vi "Load Proto File.vi"(8 "error in (no error)":errorcluster, 10 "Proto File Path":path, 11 "OOP Server in":refnum<class "Template Server.lvclass">) -> (0 "error out":errorcluster, 3 "OOP Server out":refnum<class "Template Server.lvclass">)   [LabVIEW 2019, in "Template Server.lvlib" / "Template Server.lvclass"]
uses:
  Template Server.lvclass
  typeDefs/Server gRPC UEs.ctl
  gRPC interface/Server API/typeDefs/Message Metadata.ctl
  gRPC interface/Server API/typeDefs/Message Element Metadata.ctl
  gRPC interface/Server API/typeDefs/Message Element Type.ctl
  typeDefs/Server Internal UEs.ctl
  typeDefs/Server Internal Data.ctl
  Template Server.lvclass/Template Server.ctl
  gRPC interface/gprc-lvsupport.lvlib
  gRPC interface/Server API/typeDefs/grpcId.ctl
  gRPC interface/Server API/typeDefs/gRPCId Cluster.ctl
  gRPC interface/Server API/typeDefs/gRPCId Cluster UE.ctl
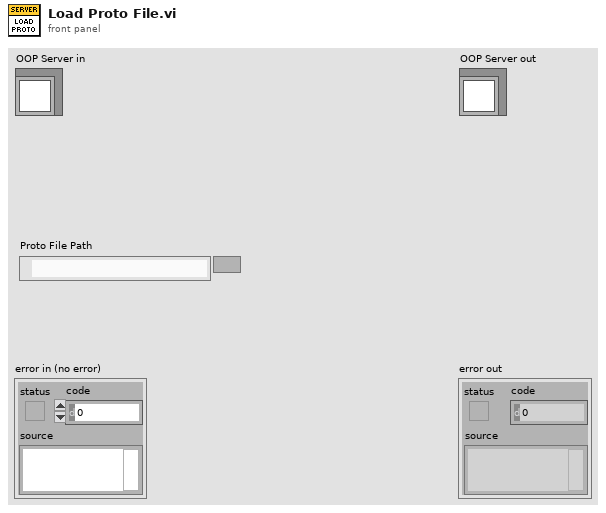
[diagram p1: front panel]
types:
  T1 = typedef "Template Server.lvlib/Template Server.lvclass/Server Internal UEs.ctl" = cluster{"Template Internal UE":refnum<user-event>}
  T2 = typedef "gprc-lvsupport.lvlib/Message Metadata.ctl" = cluster{"Name":string, "Elements":T3[]}
  T3 = typedef "gprc-lvsupport.lvlib/Message Element Metadata.ctl" = cluster{"Embedded Message Name":string, "Protobuf Index":i32, "MessageElementType":T4, "Repeated":bool}
  T4 = typedef "gprc-lvsupport.lvlib/Message Element Type.ctl" = enum32{"Int32Value", "FloatValue", "DoubleValue", "BoolValue", "StringValue", "MessageValue", ""}
  T5 = typedef "Template Server.lvlib/Template Server.lvclass/Server gRPC UEs.ctl" = cluster{"Template gRPCId UE":T6}
  T6 = typedef "gprc-lvsupport.lvlib/gRPCId Cluster UE.ctl" = refnum<user-event>
  T7 = typedef "gprc-lvsupport.lvlib/grpcId.ctl" = u64
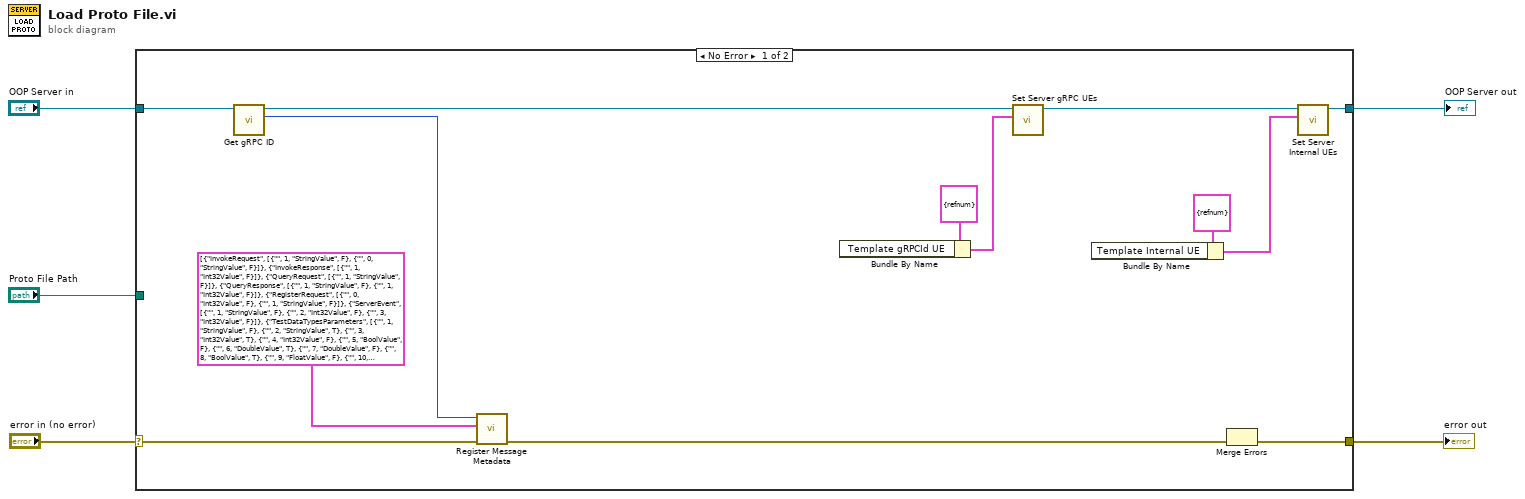
[diagram p0: block diagram]
diagram:
  n1 = case shown="No Error" "error in (no error)" {
    selector: "error in (no error)" -> [w10 w20]
    tunnel: [w6 w20] -> w4
    tunnel: [w12 w19] -> w2
    tunnel: "OOP Server in" -> [w11 w19]
    tunnel: "Proto File Path" -> [_ _]
    frame No Error {
      n2 = call "Get gRPC ID.vi"("OOP Server in"=w11) -> ("gRPC ID"=w8:T7, "OOP Server out"=w9:refnum<class "Template Server.lvclass">)  [unwired: 9 in]
      n3 = call "Register Message Metadata.vi"("error in (no error)"=w10, "Messages"=T2[] [{"Name"="InvokeRequest", "Elements"=[{"Embedded Message Name"="", "Protobuf Index"=1, "MessageElementType"=enum."StringValue", "Repeated"=FALSE}, {"Embedded Message Name"="", "Protobuf Index"=0, "MessageElementType"=enum."StringValue", "Repeated"=FALSE}]}, {"Name"="InvokeResponse", "Elements"=[{"Embedded Message Name"="", "Protobuf Index"=1, "MessageElementType"=enum."Int32Value", "Repeated"=FALSE}]}, {"Name"="QueryRequest", "Elements"=[{"Embedded Message Name"="", "Protobuf Index"=1, "MessageElementType"=enum."StringValue", "Repeated"=FALSE}]}, {"Name"="QueryResponse", "Elements"=[{"Embedded Message Name"="", "Protobuf Index"=1, "MessageElementType"=enum."StringValue", "Repeated"=FALSE}, {"Embedded Message Name"="", "Protobuf Index"=1, "MessageElementType"=enum."Int32Value", "Repeated"=FALSE}]}, {"Name"="RegisterRequest", "Elements"=[{"Embedded Message Name"="", "Protobuf Index"=0, "MessageElementType"=enum."Int32Value", "Repeated"=FALSE}, {"Embedded Message Name"="", "Protobuf Index"=1, "MessageElementType"=enum."StringValue", "Repeated"=FALSE}]}, {"Name"="ServerEvent", "Elements"=[{"Embedded Message Name"="", "Protobuf Index"=1, "MessageElementType"=enum."StringValue", "Repeated"=FALSE}, {"Embedded Message Name"="", "Protobuf Index"=2, "MessageElementType"=enum."Int32Value", "Repeated"=FALSE}, {"Embedded Message Name"="", "Protobuf Index"=3, "MessageElementType"=enum."Int32Value", "Repeated"=FALSE}]}, {"Name"="TestDataTypesParameters", "Elements"=[{"Embedded Message Name"="", "Protobuf Index"=1, "MessageElementType"=enum."StringValue", "Repeated"=FALSE}, {"Embedded Message Name"="", "Protobuf Index"=2, "MessageElementType"=enum."StringValue", "Repeated"=TRUE}, {"Embedded Message Name"="", "Protobuf Index"=3, "MessageElementType"=enum."Int32Value", "Repeated"=TRUE}, {"Embedded Message Name"="", "Protobuf Index"=4, "MessageElementType"=enum."Int32Value", "Repeated"=FALSE}, {"Embedded Message Name"="", "Protobuf Index"=5, "MessageElementType"=enum."BoolValue", "Repeated"=FALSE}, {"Embedded Message Name"="", "Protobuf Index"=6, "MessageElementType"=enum."DoubleValue", "Repeated"=TRUE}, {"Embedded Message Name"="", "Protobuf Index"=7, "MessageElementType"=enum."DoubleValue", "Repeated"=FALSE}, {"Embedded Message Name"="", "Protobuf Index"=8, "MessageElementType"=enum."BoolValue", "Repeated"=TRUE}, {"Embedded Message Name"="", "Protobuf Index"=9, "MessageElementType"=enum."FloatValue", "Repeated"=FALSE}, {"Embedded Message Name"="", "Protobuf Index"=10, "MessageElementType"=enum."FloatValue", "Repeated"=TRUE}, {"Embedded Message Name"="DataTypeTest", "Protobuf Index"=11, "MessageElementType"=enum."MessageValue", "Repeated"=FALSE}, {"Embedded Message Name"="DataTypeTest", "Protobuf Index"=12, "MessageElementType"=enum."MessageValue", "Repeated"=TRUE}]}, {"Name"="DataTypeTest", "Elements"=[{"Embedded Message Name"="", "Protobuf Index"=1, "MessageElementType"=enum."BoolValue", "Repeated"=FALSE}, {"Embedded Message Name"="", "Protobuf Index"=2, "MessageElementType"=enum."Int32Value", "Repeated"=FALSE}, {"Embedded Message Name"="", "Protobuf Index"=3, "MessageElementType"=enum."FloatValue", "Repeated"=FALSE}, {"Embedded Message Name"="", "Protobuf Index"=4, "MessageElementType"=enum."DoubleValue", "Repeated"=FALSE}]}], "gRPCid"=w8) -> ("error out"=w7:errorcluster)  [unwired: 7 in, 1 out]
      n4 = Bundle By Name(cluster=T5 {"Template gRPCId UE"=refnum} ("gRPC Server Method Events")) -> (w16:T5)  [unwired: 1 in]
      n5 = call "Set Server gRPC UEs.vi"("Server gRPC UEs"=w16, "OOP Server in"=w9) -> ("OOP Server out"=w15:refnum<class "Template Server.lvclass">)  [unwired: 9 in]
      n6 = Bundle By Name(cluster=T1 {"Template Internal UE"=refnum} ("Server Internal UEs")) -> (w13:T1)  [unwired: 1 in]
      n7 = Merge Errors(w7) -> (w6:errorcluster)  [unwired: 1 in]
      n8 = call "Set Server Internal UEs.vi"("Server Internal UEs"=w13, "OOP Server in"=w15) -> ("OOP Server out"=w12:refnum<class "Template Server.lvclass">)  [unwired: 9 in]
    }
    frame Error {
    }
  }
  "error out" <- w4
  "OOP Server out" <- w2
